vi "Test2_3b_ASIC.vi"(0 "Instrument VISA in":T1={"AWG VISA"="generadorpulsos", "Oscilloscope  VISA "="Oscilloscope", "Integration Board IP"="172.16.7.43", "connection ID"=refnum, "report out"=refnum, "report file path"=path "C:/Documents and Settings/CTA_LAB01/Desktop/L0_Asic/L0 Asic Test Data"}, 1 "Serial Number":string="SN023", 5 "quantity":i32=2, 7 "Cycles Burst":i32=10000, 9 "L1 Address":i32=17, 11 "error in":errorcluster={"status"=TRUE, "code"=-1074000000, "source"="Agilent 8000 Series.lvlib:Error Query.vi<ERR>\nInstrument reports:\n-410,\"Query INTERRUPTED\"\r\n0,\"No error\"\r\n\n\n\n<b>Complete call chain:</b>\r\n     Agilent 8000 Series.lvlib:Error Query.vi\r\n     Agilent 8000 Series.lvlib:Close.vi\r\n     Test2_3a_ASIC.vi\r\n     Test_Sum_plus_Maj.vi"}, 12 "channel array":i32[](array[numeric])=[0, 1, 2, 3, 4, 5, 6]) -> (4 "Instrument VISA out":T1={"AWG VISA"="", "Oscilloscope  VISA "="", "Integration Board IP"="", "connection ID"=refnum, "report out"=refnum, "report file path"=path "C:/Documents and Settings/CTA_LAB01/Desktop/L0_Asic/L0 Asic Test Data"}, 15 "error out":errorcluster={"status"=TRUE, "code"=63, "source"="TCP Open Connection in Test2_3b_ASIC.vi"})   [LabVIEW 2009]
uses:
  <vilib>/Utility/NIReport.llb/NI_report.lvclass
  <instrlib>/Agilent 81150/Agilent 81150.lvlib
  L0_Asic/L0 Asic Test Folder v9/C/Program Files/National Instruments/LabVIEW 2012/instr.lib/Agilent 8000 Series/Agilent 8000 Series.lvlib
panel:
  out "Array":i32[](array[numeric])=[2, 3, 5]
  out "points quantity":dbl=94.0
  out "appended array":dbl[](array[numeric])=[0.75, 42.0, 0.0, 63.0, 1.0, 1.069, 0.0055, 2.925838e-09, 1.2702e-11, 0.0555, 0.0035, 9.99999e+37, 9.99999e+37, 6.264189e-09, 3.2805e-11, 94.0]
  out "read buffer 3":string="V amptd(f2),1.074E+00,0,1.056E+00,1.087E+00,1.0690E+00,5.5E-03,9.4E+01,+ width(f2),2.90015E-09,0,2.90015E-09,2.95960E-09,2.925838E-09,1.2702E-11,9.4E+01,V amptd(1),5.5E-02,0,4.8E-02,6.7E-02,5.55E-02,3.5E-03,9.4E+01,+ width(f1),9.99999E+37,5,9.99999E+37,9.99999E+37,9.99999E+37,9.99999E+37,9.99999E+37,Time(f1-f2),6.26722E-09,0,6.20145E-09,6.35270E-09,6.264189E-09,3.2805E-11,9.4E+01\n"
  in  "Quantity of measurements":u32=100
  in  "Voltage":dbl[](array[numeric])=[0.05, 0.1, 0.2, 0.5, 0.8]
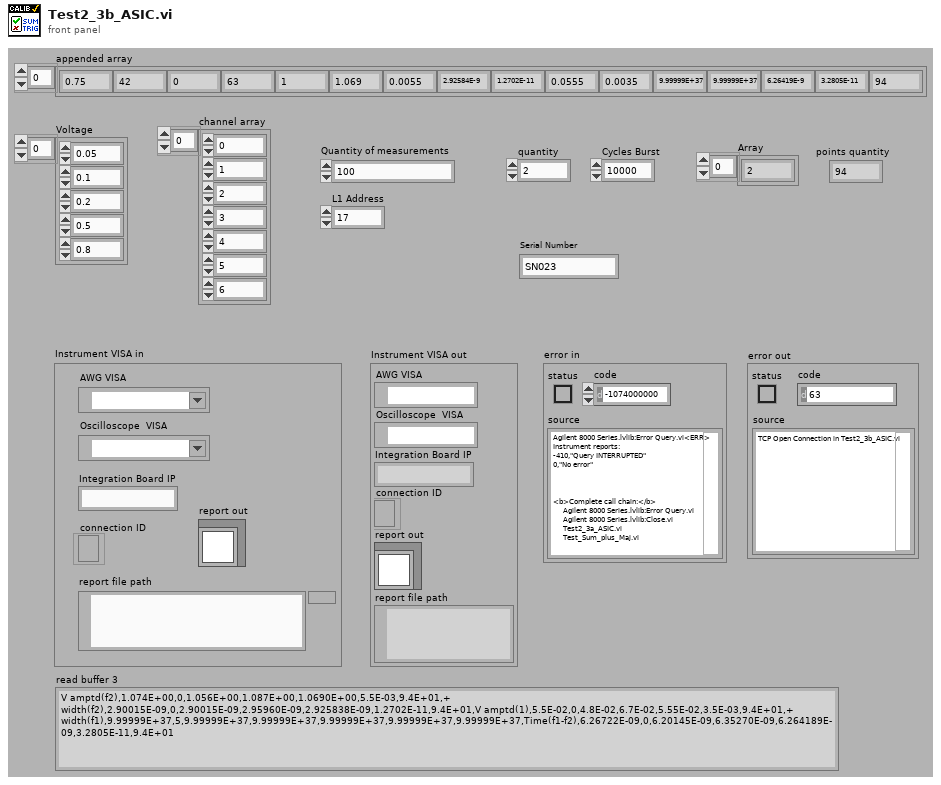
[diagram p1: front panel]
types:
  T1 = cluster{"AWG VISA":refnum<visa-resource-name>, "Oscilloscope  VISA ":refnum<visa-resource-name>, "Integration Board IP":string, "connection ID":refnum<k5>, "report out":refnum<class "NI_report.lvclass">, "report file path":path}
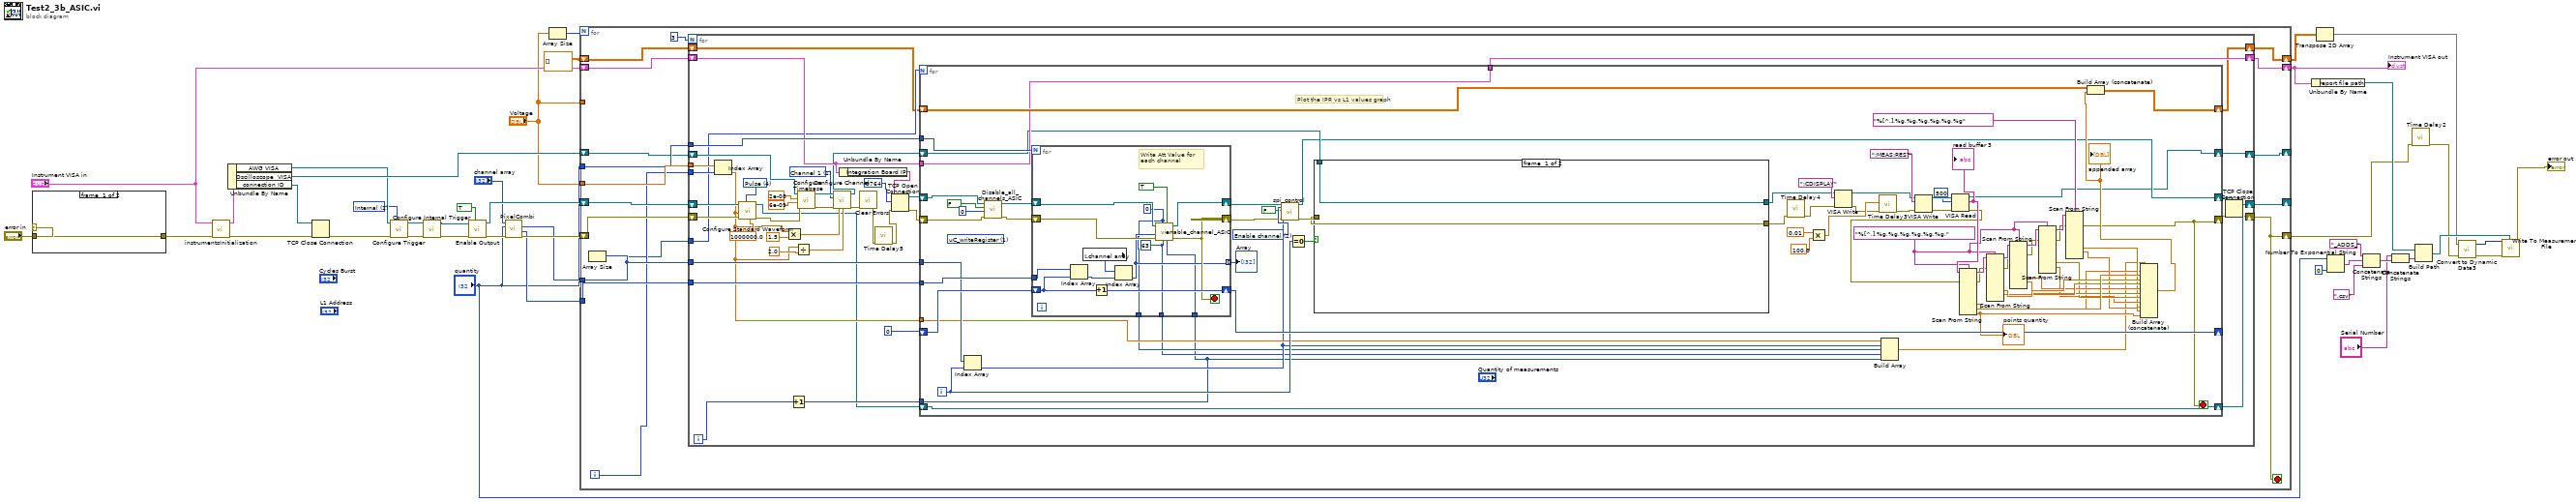
[diagram p0: block diagram]
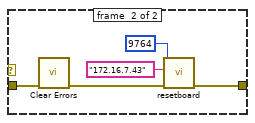
[diagram p2: hidden frame]
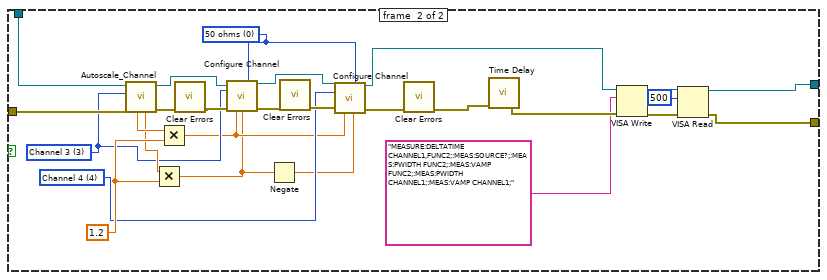
[diagram p3: hidden frame]
diagram:
  w11 = u16 1 items=["Immediate", "Internal", "External", "Software Trigger Function"] ("Trigger Source (0: Immediate)")
  n1 = case shown="Error" "error in" {
    tunnel: "error in" -> [w42 w44]
    tunnel: [w42 w47] -> w7
    frame #0 {
    }
    frame #1 {
      n2 = call <vilib>:"Clear Errors.vi"("error in (no error)"=w44) -> ("error out"=w43:errorcluster)  [unwired: 6 in]
      n3 = call "resetboard.vi"("error in (no error)"=w43, "address"="172.16.7.43", "remote port or service name"=u16 9764) -> ("error out"=w47:errorcluster)  [unwired: 7 in, 1 out]
    }
  }
  n4 = call "instrumentsInitialization.vi"("error in"=w7, "Instrument VISA in"="Instrument VISA in") -> ("error out"=w5:errorcluster, "Instrument VISA out"=w30:T1)  [unwired: 8 in]
  n5 = Unbundle By Name(w30) -> ("AWG VISA"=w14:refnum<visa-resource-name>, "Oscilloscope  VISA"=w29:refnum<visa-resource-name>, "connection ID"=w6:refnum<k5>)
  n6 = TCP Close Connection(connection ID=w6, error in (no error)=w5) -> (error out=w4:errorcluster)  [unwired: 1 in, 1 out]
  n7 = call <instrlib>:"Configure Trigger.vi"("Trigger Source (0: Immediate)"=w11, "error in (no error)"=w4, "VISA resource name"=w14) -> ("error out"=w12:errorcluster, "VISA resource name out"=w13:refnum<visa-resource-name>)  [unwired: 7 in]
  n8 = call <instrlib>:"Configure Internal Trigger.vi"("error in (no error)"=w12, "VISA resource name"=w13) -> ("error out"=w15:errorcluster, "VISA resource name out"=w16:refnum<visa-resource-name>)  [unwired: 8 in]
  n9 = call <instrlib>:"Enable Output.vi"("Enable Output (T: Enable)"=TRUE, "error in (no error)"=w15, "VISA resource name"=w16) -> ("error out"=w40:errorcluster, "VISA resource name out"=w38:refnum<visa-resource-name>)  [unwired: 7 in]
  n10 = call "PixelCombi.vi"("error in"=w40, "quantity"="quantity", "array"="channel array") -> ("error out"=w39:errorcluster, "Channels"=w37:i32[], "Combination Array"=w36:i16[])  [unwired: 6 in]
  n11 = Array Size(array="Voltage") -> (size(s)=w31:i32)
  n12 = for {
    N: w31 -> [_]
    tunnel: w37 -> [w62]
    tunnel: w36 -> [w61]
    shift-right: [w48] -> w18
    shift-left: w39 -> [w64]
    tunnel: "Voltage" -> [w60]
    tunnel: "Voltage" -> [_]
    tunnel: "quantity" -> [w58]
    shift-right: [w53] -> w17
    shift-left: "Instrument VISA in" -> [w56]
    shift-right: [w52] -> w21
    shift-left: dbl[][] [] -> [w54]
    shift-right: [w49] -> _
    shift-left: w38 -> [w63]
    shift-right: [w50] -> _
    shift-left: w29 -> [w57]
    i -> [w59]
    stop <- w48 stop-if-true
    n13 = Array Size(array=w61) -> (size(s)=w55:i32)
    n14 = for {
      N: 3 -> [_]
      tunnel: w62 -> [w103]
      tunnel: w61 -> [w101]
      tunnel: w60 -> [w100]
      tunnel: w59 -> [w99]
      tunnel: w58 -> [w98]
      tunnel: w55 -> [w83]
      shift-right: [w73] -> w52
      shift-left: w54 -> [w76]
      shift-right: [w74] -> w53
      shift-left: w56 -> [w87]
      shift-right: [w68] -> w48
      shift-left: w64 -> [w105]
      shift-right: [w69] -> w49
      shift-left: w63 -> [w104]
      shift-right: [w71] -> w50
      shift-left: w57 -> [w94]
      i -> [w65]
      w90 = 1 items=["Channel 1"=1, "Channel 2"=2, "Channel 3"=3, "Channel 4"=4] ("Channel (1: Channel 1)")
      w107 = u16 4 items=["Sine", "Square", "Ramp Up", "Ramp Down", "Pulse", "Noise", "DC"] ("Waveform (0: Sine)")
      n15 = Index Array(array=w100, index=w99) -> (element=w75:dbl)
      n16 = call <instrlib>:"Configure Standard Waveform.vi"("Frequency (1000.0 Hz)"=1000000.0, "Waveform (0: Sine)"=w107, "error in (no error)"=w105, "Amplitude (1.0 Vpp)"=w75, "VISA resource name"=w104) -> ("error out"=w97:errorcluster, "VISA resource name out"=w70:refnum<visa-resource-name>)  [unwired: 5 in]
      n17 = Multiply(x=w75, y=1.5) -> (x*y=w89:dbl)
      n18 = Increment(x=w65) -> (x+1=w72:i32)
      n19 = Divide(x=w75, y=2.0) -> (x/y=w81:dbl)
      n20 = call <instrlib>:"Configure Timebase.vi"("error in (no error)"=w97, "Position (0.0 s)"=6e-09, "Timebase (0.005 s)"=2e-08, "VISA resource name"=w94) -> ("error out"=w96:errorcluster, "VISA resource name out"=w93:refnum<visa-resource-name>)  [unwired: 6 in]
      n21 = call "Configure Channel.vi"("VISA resource name"=w93, "Channel (1: Channel 1)"=w90, "error in (no error)"=w96, "Vertical Range (2.0 V)"=w89, "Vertical Offset (0.0 V)"=w81) -> ("VISA resource name out"=w80:refnum<visa-resource-name>, "error out"=w95:errorcluster)  [unwired: 9 in]
      n22 = Unbundle By Name(w87) -> ("Integration Board IP"=w85:string)
      n23 = call <vilib>:"Clear Errors.vi"("error in (no error)"=w95) -> ("error out"=w67:errorcluster)  [unwired: 6 in]
      n24 = call "Time Delay5"("error in (no error)"=w67) -> ("error out"=w66:errorcluster)  [unwired: 10 in]
      n25 = TCP Open Connection(address=w85, remote port or service name=u16 9764, error in (no error)=w66) -> (connection ID=w77:refnum<k5>, error out=w86:errorcluster)  [unwired: 2 in]
      n26 = for {
        N: w83 -> [_]
        tunnel: w101 -> [w175]
        tunnel: w103 -> [w176]
        shift-right: [w177] -> _
        shift-left: i16 0 ("element") -> [w178]
        shift-right: [w122] -> w79
        shift-left: w86 -> [w168]
        tunnel: w87 -> [w163]
        tunnel: w98 -> [w174]
        tunnel: [w163] -> w74
        shift-right: [w169] -> w73
        shift-left: w76 -> [w170]
        shift-right: [w123] -> w78
        shift-left: w77 -> [w121]
        tunnel: w75 -> [w118]
        tunnel: w72 -> [w113]
        shift-right: [w112] -> w71
        shift-left: w80 -> [w161]
        shift-right: [w111] -> w69
        shift-left: w70 -> [w111]
        i -> [w159]
        stop <- w122 stop-if-true
        w144 = "%[^,],%g,%g,%g,%g,%g,%g," ("format string")
        w167 = u16 2 items=["Attenuation", "Clipping", "Enable channel", "Delay line", "ASIC"] ("Device")
        (unwired) u16 1 items=["sendCommand"=9, "FPGA_writeRegister"=3, "FPGA_readRegister"=2, "uC_writeRegister"=1, "uC_readRegister"=0] ("Action")
        # "Plot the IPR vs L1 values graph"
        n27 = Index Array(array=w175, index=w159) -> (element=w117:i16)
        n28 = call "Disable_all_channels_ASIC.vi"("error in"=w168, "id_in"=0 ("Data"), "Clip_en_b"=FALSE, "connection ID"=w121) -> ("error out"=w172:errorcluster, "connection ID out"=w171:refnum<k5>)  [unwired: 5 in, 1 out]
        n29 = for {
          N: w174 -> [_]
          shift-right: [w220] -> w177
          shift-left: w178 -> [w221]
          tunnel: w176 -> [w219]
          shift-right: [w216] -> w165
          shift-left: w172 -> [w215]
          shift-right: [w213] -> w164
          shift-left: w171 -> [w214]
          tunnel: [w212] -> w120 mode=indexing
          tunnel: [w211] -> w116
          tunnel: [w210] -> w115
          tunnel: w113 -> [w209]
          stop <- w216 stop-if-true
          w211 = u32 0 ("Att gain")
          w210 = u32 63 ("Ib_clipVb")
          # "Write Att Value for each channel"
          n30 = Index Array(array=w219, index=w221) -> (element=w217:i32)
          n31 = local read "channel array"() -> (w218:i32[])
          n32 = Increment(x=w221) -> (x+1=w220:i16)
          n33 = Index Array(array=w218, index=w217) -> (element=w212:i32)
          n34 = call "enable_channel_ASIC.vi"("Clip_sel_b"=w209, "maj/sum"=TRUE, "Ib_clipVb"=w210, "Att gain"=w211, "error in"=w215, "Channel"=w212, "connection ID"=w214) -> ("error out"=w216:errorcluster, "connection ID out"=w213:refnum<k5>)  [unwired: 2 in, 1 out]
        }
        "Array" <- w120
        n35 = call "spi_control.vi"("connection ID"=w164, "Device"=w167, "Read/#write"=FALSE, "Data"=w117, "error out 3"=w165) -> ("connection ID out"=w123:refnum<k5>, "error out 2"=w162:errorcluster)  [unwired: 7 in, 6 out]
        n36 = Equal To 0?(x=w159) -> (x = 0?=w160:bool)
        n37 = case shown="True" w160 {
          tunnel: [w180 w187] -> w108
          tunnel: w162 -> [w180 w193]
          tunnel: w161 -> [w179 w194]
          tunnel: [w179 w196] -> w126
          frame #0 {
          }
          frame #1 {
            w197 = u32 0 items=["50 ohms", "1 Mohms"] ("Input Impedance (1: 1 Mohms)")
            w185 = 3 items=["Channel 1"=1, "Channel 2"=2, "Channel 3"=3, "Channel 4"=4] ("Channel (1: Channel 1)")
            w184 = 4 items=["Channel 1"=1, "Channel 2"=2, "Channel 3"=3, "Channel 4"=4] ("Channel (1: Channel 1)")
            w190 = 1.2 ("y")
            n38 = call "Autoscale_Channel.vi"("error in"=w193, "Channel"=w185, "VISA resource name"=w194) -> ("error out"=w204:errorcluster, "VISA resource name out"=w207:refnum<visa-resource-name>, "Offset"=w186:dbl, "VerticalRange"=w201:dbl)  [unwired: 5 in]
            n39 = Multiply(x=w186, y=w190) -> (x*y=w182:dbl)
            n40 = Multiply(x=w201, y=w190) -> (x*y=w183:dbl)
            n41 = call <vilib>:"Clear Errors.vi"("error in (no error)"=w204) -> ("error out"=w205:errorcluster)  [unwired: 6 in]
            n42 = call "Configure Channel.vi"("VISA resource name"=w207, "Input Impedance (1: 1 Mohms)"=w197, "Channel (1: Channel 1)"=w185, "error in (no error)"=w205, "Vertical Range (2.0 V)"=w183, "Vertical Offset (0.0 V)"=w182) -> ("VISA resource name out"=w202:refnum<visa-resource-name>, "error out"=w206:errorcluster)  [unwired: 8 in]
            n43 = Negate(x=w182) -> (-x=w181:dbl)
            n44 = call <vilib>:"Clear Errors.vi"("error in (no error)"=w206) -> ("error out"=w195:errorcluster)  [unwired: 6 in]
            n45 = call "Configure Channel.vi"("VISA resource name"=w202, "Input Impedance (1: 1 Mohms)"=w197, "Channel (1: Channel 1)"=w184, "error in (no error)"=w195, "Vertical Range (2.0 V)"=w183, "Vertical Offset (0.0 V)"=w181) -> ("VISA resource name out"=w191:refnum<visa-resource-name>, "error out"=w203:errorcluster)  [unwired: 8 in]
            n46 = call <vilib>:"Clear Errors.vi"("error in (no error)"=w203) -> ("error out"=w192:errorcluster)  [unwired: 6 in]
            n47 = call "Time Delay"("error in (no error)"=w192) -> ("error out"=w189:errorcluster)  [unwired: 10 in]
            n48 = VISA Write(VISA resource name=w191, write buffer="MEASURE:DELTATIME CHANNEL1,FUNC2;:MEAS:SOURCE?;:MEAS:PWIDTH FUNC2;:MEAS:VAMP FUNC2;:MEAS:PWIDTH CHANNEL1;:MEAS:VAMP CHANNEL1;", error in (no error)=w189) -> (VISA resource name out=w200:refnum<visa-resource-name>, error out=w199:errorcluster)  [unwired: 1 out]
            n49 = VISA Read(VISA resource name=w200, byte count=u32 500, error in (no error)=w199) -> (VISA resource name out=w196:refnum<visa-resource-name>, error out=w187:errorcluster)  [unwired: 2 out]
          }
        }
        n50 = call "Time Delay4"("error in (no error)"=w108) -> ("error out"=w109:errorcluster)  [unwired: 10 in]
        n51 = Multiply(x=0.01, y=100.0) -> (x*y=w151:dbl)
        n52 = VISA Write(VISA resource name=w126, write buffer=":CDISPLAY", error in (no error)=w109) -> (VISA resource name out=w129:refnum<visa-resource-name>, error out=w127:errorcluster)  [unwired: 1 out]
        n53 = call "Time Delay3"("error in (no error)"=w127, "Delay Time (s)"=w151) -> ("error out"=w150:errorcluster)  [unwired: 9 in]
        n54 = Build Array(w118, w117, w116, w115, w113) -> (w114:dbl[])
        n55 = VISA Write(VISA resource name=w129, write buffer=":MEAS:RES?", error in (no error)=w150) -> (VISA resource name out=w158:refnum<visa-resource-name>, error out=w157:errorcluster)  [unwired: 1 out]
        n56 = VISA Read(VISA resource name=w158, byte count=u32 500, error in (no error)=w157) -> (VISA resource name out=w112:refnum<visa-resource-name>, read buffer=w154:string, error out=w134:errorcluster)  [unwired: 1 out]
        "read buffer 3" <- w154
        n57 = Scan From String(format string=w144, input string=w154, error in=w134) -> (remaining string=w148:string, error out=w130:errorcluster, output 5=w119:dbl, output 6=w149:dbl, output 7=w135:dbl)  [unwired: 12 in, 1 out]
        "points quantity" <- w135
        n58 = Scan From String(format string=w144, input string=w148, error in=w130) -> (remaining string=w145:string, error out=w131:errorcluster, output 5=w142:dbl, output 6=w141:dbl)  [unwired: 13 in, 1 out]
        n59 = Scan From String(format string=w144, input string=w145, error in=w131) -> (remaining string=w146:string, error out=w132:errorcluster, output 5=w140:dbl, output 6=w139:dbl)  [unwired: 13 in, 1 out]
        n60 = Scan From String(format string=w144, input string=w146, error in=w132) -> (remaining string=w147:string, error out=w133:errorcluster, output 5=w138:dbl, output 6=w137:dbl)  [unwired: 13 in, 1 out]
        n61 = Scan From String(format string="%[^,],%g,%g,%g,%g,%g,%g", input string=w147, error in=w133) -> (error out=w122:errorcluster, output 5=w125:dbl, output 6=w136:dbl)  [unwired: 13 in, 2 out]
        n62 = Build Array (concatenate)(w114, w119, w149, w142, w141, w140, w139, w138, w137, w125, w136, w135) -> (w124:dbl[])
        "appended array" <- w124
        n63 = Build Array (concatenate)(w170, w124) -> (w169:dbl[][])
      }
      n64 = TCP Close Connection(connection ID=w78, error in (no error)=w79) -> (error out=w68:errorcluster)  [unwired: 1 in, 1 out]
    }
  }
  "Instrument VISA out" <- w17
  n65 = Unbundle By Name(w17) -> ("report file path"=w34:path)
  n66 = Transpose 2D Array(2D array=w21) -> (transposed array=w9:dbl[][])
  n67 = Number To Exponential String(number="quantity", precision (6)=i16 0) -> (E-format string=w25:string)  [unwired: 2 in]
  n68 = Concatenate Strings("_ADDS_" ("string"), w25, ".csv" ("name or relative path")) -> (w2:string)
  n69 = Concatenate Strings("Serial Number", w2) -> (w3:string)
  n70 = call "Time Delay2"("error in (no error)"=w18) -> ("error out"=w32:errorcluster)  [unwired: 10 in]
  n71 = Build Path(base path=w34, name or relative path=w3) -> (appended path=w33:path)
  n72 = call "Convert to Dynamic Data3"("2D Array"=w9) -> ("Dynamic Data Type"=w10:dynamicdata)  [unwired: 3 in]
  n73 = call "Write To Measurement File"("Signals"=w10, "error in (no error)"=w32, "Filename"=w33) -> ("error out"=→"error out":errorcluster)  [unwired: 14 in, 2 out]
